vi "Write Assign Instrument.vi"(10 "Assign Instrument":T2, 11 "Test Framework in":refnum<class "Test Framework.lvclass">) -> (3 "Test Framework out":refnum<class "Test Framework.lvclass">)   [LabVIEW 2020, in "Test Framework.lvclass"]
uses:
  Test Framework.lvclass
  Controls/Reference Selector.ctl
  Test Framework.lvclass/Test Framework.ctl
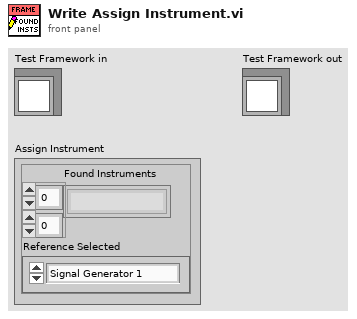
[diagram p1: front panel]
types:
  T1 = typedef "Test Framework.lvclass/Reference Selector.ctl" = enum16{"Signal Generator 1", "Signal Generator 2", "Spectrum Analyzer"}
  T2 = cluster{"Found Instruments":string[][], "Reference Selected":T1}
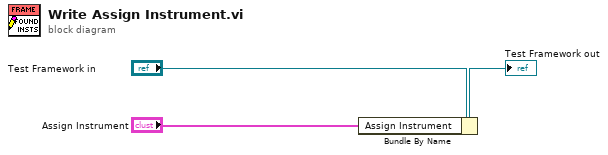
[diagram p0: block diagram]
diagram:
  n1 = Bundle By Name(cluster="Test Framework in", "Assign Instrument"="Assign Instrument") -> (→"Test Framework out":refnum<class "Test Framework.lvclass">)
